vi "RPi_BME280_Registers_to_Raw_Measures_Conversion.vi"(0 "Registers (Bytes)":u8[](array[numeric])) -> (4 "Raw Measures":T1)   [LabVIEW 2020]
doc: "Converts Registers to Raw Pressure, Temperature and Humidity Measures\n\nMIT License\nCopyright (c) 2021 Asper"
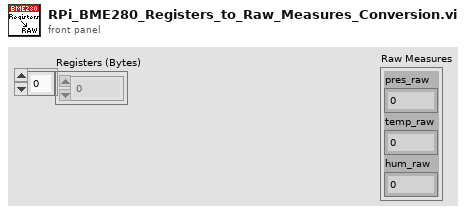
[diagram p1: front panel]
types:
  T1 = cluster{"pres_raw":u32, "temp_raw":u32, "hum_raw":u32}
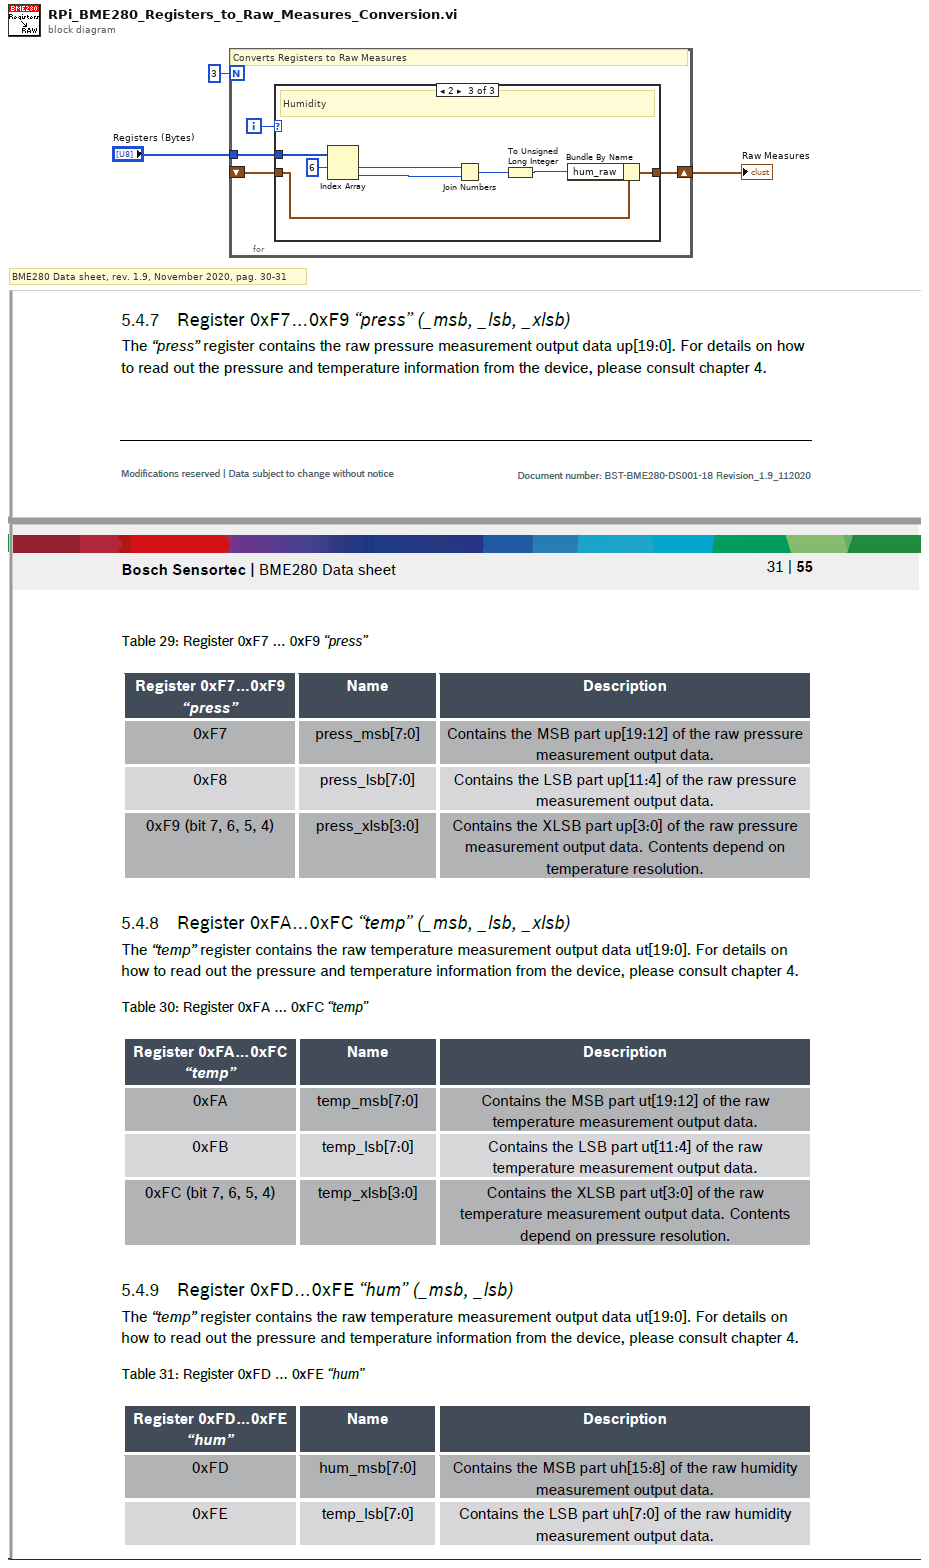
[diagram p0: block diagram]
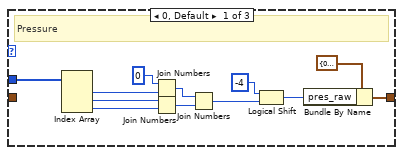
[diagram p2: hidden frame]
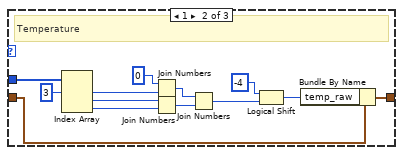
[diagram p3: hidden frame]
diagram:
  # "BME280 Data sheet, rev. 1.9, November 2020, pag. 30-31"
  n1 = for {
    N: 3 -> [_]
    tunnel: "Registers (Bytes)" -> [w7]
    shift-right: [w5] -> w2
    shift-left: _ -> [w4]
    i -> [w6]
    # "Converts Registers to Raw Measures"
    n2 = case shown="2" w6 {
      tunnel: w7 -> [w19 w32 w40]
      tunnel: [w8 w22 w38] -> w5
      tunnel: w4 -> [_ w20 w36]
      frame 0, Default {
        # "Pressure"
        n3 = Index Array(array=w19) -> (element #1=w14:u8, element #2=w13:u8, element #3=w12:u8)  [unwired: 3 in]
        n4 = Join Numbers(hi=u8 0, lo=w14) -> ((hi.lo)=w17:u16)
        n5 = Join Numbers(hi=w13, lo=w12) -> ((hi.lo)=w11:u16)
        n6 = Join Numbers(hi=w17, lo=w11) -> ((hi.lo)=w16:u32)
        n7 = Logical Shift(y=i16 -4, x=w16) -> (x << y=w10:u32)
        n8 = Bundle By Name(cluster=T1 {"pres_raw"=0, "temp_raw"=0, "hum_raw"=0}, "pres_raw"=w10) -> (w8:T1)
      }
      frame 1 {
        # "Temperature"
        n9 = Index Array(array=w32, index #1=3 ("index")) -> (element #1=w27:u8, element #2=w26:u8, element #3=w25:u8)  [unwired: 2 in]
        n10 = Join Numbers(hi=u8 0, lo=w27) -> ((hi.lo)=w30:u16)
        n11 = Join Numbers(hi=w26, lo=w25) -> ((hi.lo)=w24:u16)
        n12 = Join Numbers(hi=w30, lo=w24) -> ((hi.lo)=w29:u32)
        n13 = Logical Shift(y=i16 -4, x=w29) -> (x << y=w23:u32)
        n14 = Bundle By Name(cluster=w20, "temp_raw"=w23) -> (w22:T1)
      }
      frame 2 {
        # "Humidity"
        n15 = Index Array(array=w40, index #1=6 ("index")) -> (element #1=w35:u8, element #2=w34:u8)  [unwired: 1 in]
        n16 = Join Numbers(hi=w35, lo=w34) -> ((hi.lo)=w39:u16)
        n17 = To Unsigned Long Integer(number=w39) -> (unsigned 32bit integer=w33:u32)
        n18 = Bundle By Name(cluster=w36, "hum_raw"=w33) -> (w38:T1)
      }
    }
  }
  "Raw Measures" <- w2
